vi "NonLinearCancellation_Analysis.vi"() -> ()   [LabVIEW 2022 SP3]
uses:
  <vilib>/Analysis/baseanly.llb/Mean (DBL).vi
  <vilib>/Analysis/NI_AALBase.lvlib
panel:
  out "EOF?":bool
  in  "x0":dbl
  in  "Scaling Factor":dbl
  in  "Error":dbl
  out "XY Graph":cluster{dbl[], dbl[]}[](graph)
  out "Waveform Chart 2":dynamicdata(graph)
  out "Waveform Chart":dynamicdata(graph)
  in  "stop":bool
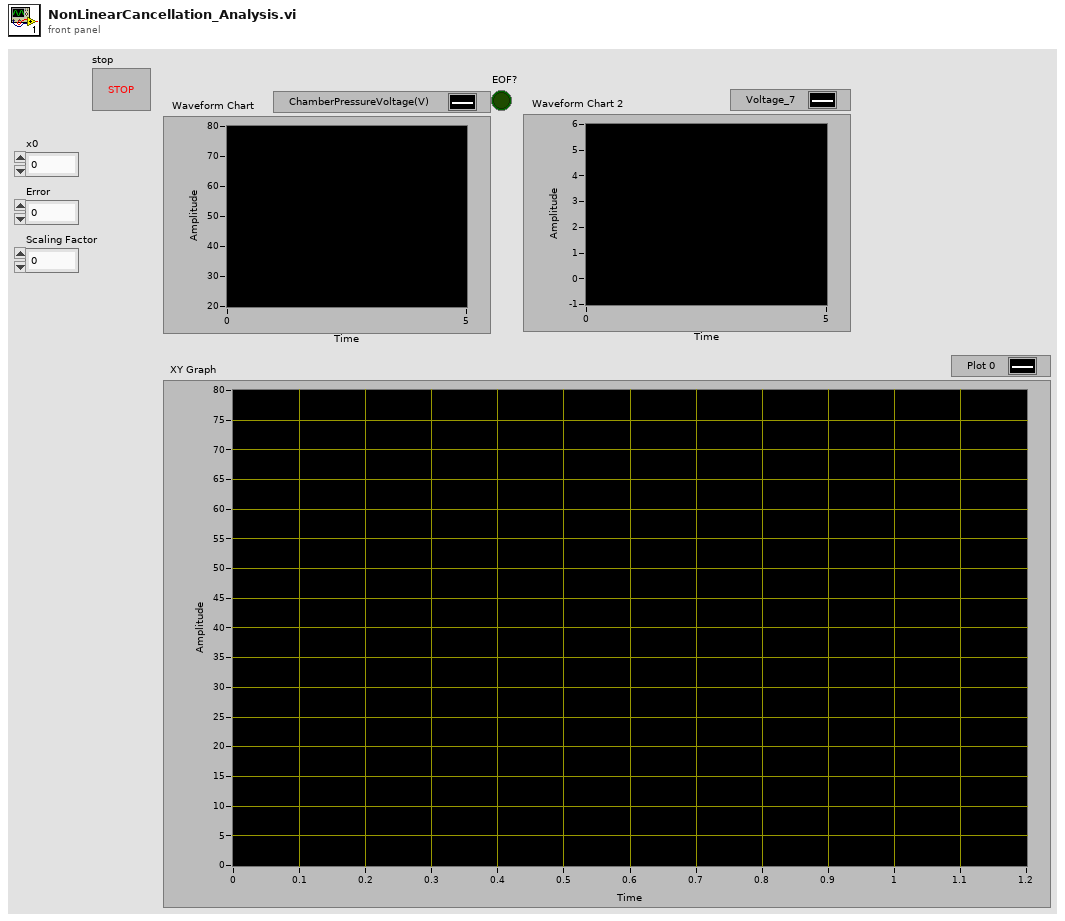
[diagram p1: front panel]
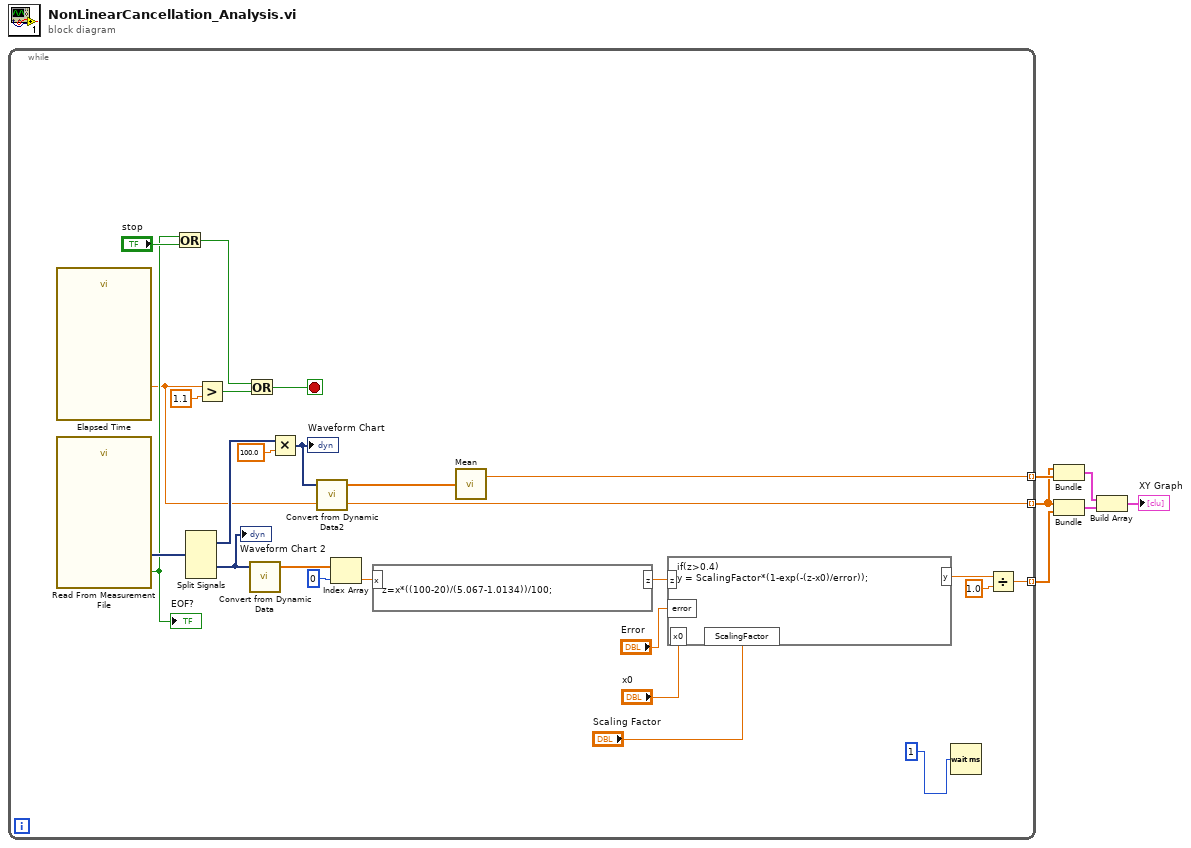
[diagram p0: block diagram]
diagram:
  n1 = while {
    tunnel: [w30] -> w6 mode=indexing
    tunnel: [w22] -> w3 mode=indexing
    tunnel: [w11] -> w4 mode=indexing
    stop <- w8 stop-if-true
    n2 = call "Elapsed Time"() -> ("Elapsed Time (s)"=w11:dbl)  [unwired: 12 in, 7 out]
    n3 = call "Read From Measurement File"() -> ("Signals"=w31:dynamicdata, "EOF?"=w13:bool)  [unwired: 6 in, 4 out]
    "EOF?" <- w13
    n4 = Or(x=w13, y="stop") -> (x .or. y?=w9:bool)
    n5 = Split Signals(w31) -> (w16:dynamicdata, w21:dynamicdata)  [unwired: 6 in, 4 out]
    "Waveform Chart 2" <- w21
    n6 = Greater?(x=w11, y=1.1) -> (0:w10:bool)
    n7 = Or(x=w9, y=w10) -> (x .or. y?=w8:bool)
    n8 = call "Convert from Dynamic Data"("Dynamic Data Type"=w21) -> ("Array"=w29:dbl[])  [unwired: 3 in]
    n9 = Multiply(x=w16, y=100.0) -> (x*y=w15:dynamicdata)
    "Waveform Chart" <- w15
    n10 = call "Convert from Dynamic Data2"("Dynamic Data Type"=w15) -> ("Array"=w20:dbl[])  [unwired: 3 in]
    n11 = Index Array(array=w29, index=0) -> (element=w19:dbl)
    n12 = formula code="z=x*((100-20)/(5.067-1.0134))/100;"("x"=w19) -> ("z"=w18:dbl)
    n13 = call-poly <vilib>:"Mean.vi"("X"=w20) -> ("mean"=w30:dbl)  [unwired: 1 out]
    n14 = formula code="if(z>0.4)\ny = ScalingFactor*(1-exp(-(z-x0)/error));"("z"=w18, "error"="Error", "ScalingFactor"="Scaling Factor", "x0"="x0") -> ("y"=w24:dbl)
    n15 = Wait (ms)(milliseconds to wait=u32 1) -> ()  [unwired: 1 out]
    n16 = Divide(x=w24, y=1.0) -> (x/y=w22:dbl)
  }
  n17 = Bundle(w4, w6) -> (w5:cluster{dbl[], dbl[]})  [unwired: 1 in]
  n18 = Bundle(w4, w3) -> (w2:cluster{dbl[], dbl[]})  [unwired: 1 in]
  n19 = Build Array(w5, w2) -> (→"XY Graph":cluster{dbl[], dbl[]}[])
